vi "Senden-01-17.vi"(5 "error in":errorcluster, 6 "BefehlsCluster":T1, 7 "AbfragenCluster":cluster{string[], string[], string[]}, 8 "Abfragenr.Cluster":cluster{i32, i32, i32}, 9 "Senden?":bool[](array[boolean]), 10 "FPGA VI Reference In":refnum<k20>) -> (0 "BefehlsCluster":T1, 2 "error out":errorcluster, 3 "Senden?":bool[](array[boolean]), 4 "Abfragenr.Cluster":cluster{i32, i32, i32})   [LabVIEW 2010]
uses:
  <vilib>/rvi/interface/nirviMethod/nirviMethod.xnode
  C:/Users/HAGAR-IV/Desktop/Zeugs/markus/version feb 2012/FPGA Bitfiles/pertrasgcfpga2_FPGATarget_FPGA-Programm-01_A75D3647.lvbitx
  C:/Users/HAGAR-IV/Desktop/Zeugs/Johnny/pertrasgc fpga/FPGA-Programm-01-17.vi
  <vilib>/rvi/interface/common/niFpgaNodeNameForErrorReporting.ctl
  <vilib>/rvi/errors/niLvFpgaWhatHappensToTopLevelVI.ctl
  <vilib>/Utility/error.llb/Error Cluster From Error Code.vi
  <vilib>/rvi/errors/niLvFpgaAdjustHostInterfaceError.vi
  NiFpgaLv.dll
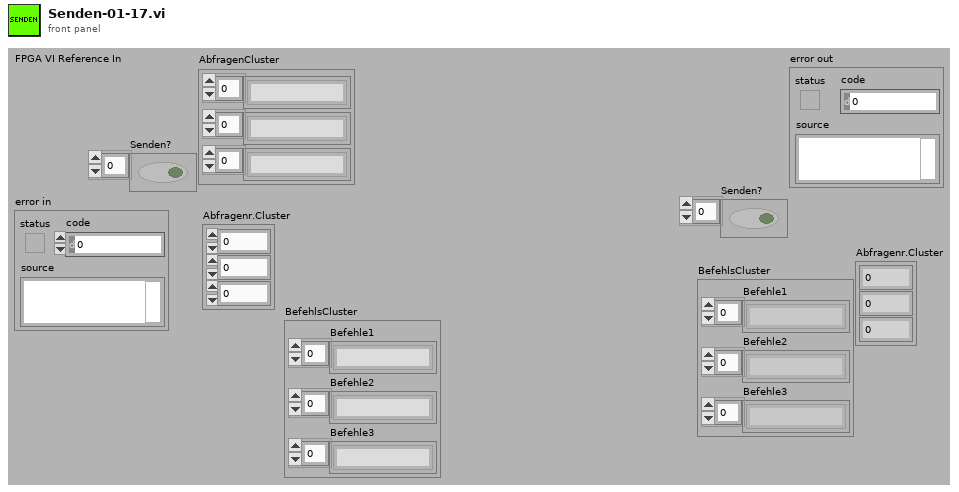
[diagram p1: front panel]
types:
  T1 = cluster{"Befehle1":string[], "Befehle2":string[], "Befehle3":string[]}
  T2 = typedef "niFpgaNodeNameForErrorReporting.ctl" = enum16{"Open FPGA VI Reference", "Read/Write Control", "Invoke Method: Abort", "Invoke Method: Acknowledge IRQ", "Invoke Method: Download", "Invoke Method: FIFO.Configure", "Invoke Method: FIFO.Read", "Invoke Method: FIFO.Start", "Invoke Method: FIFO.Stop", "Invoke Method: FIFO.Write", "Invoke Method: Reset", "Invoke Method: Run", "Invoke Method: Wait on IRQ", "Close FPGA VI Reference"}
  T3 = typedef "niLvFpgaWhatHappensToTopLevelVI.ctl" = enum16{"top level VI scripted behind XNode", "top level VI inlined behind XNode"}
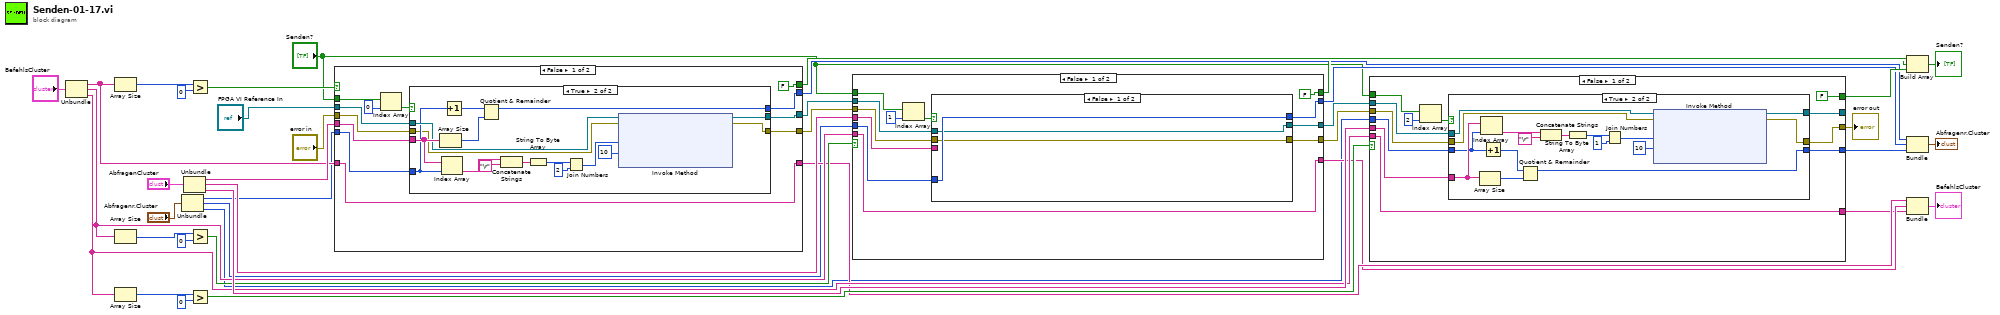
[diagram p0: block diagram]
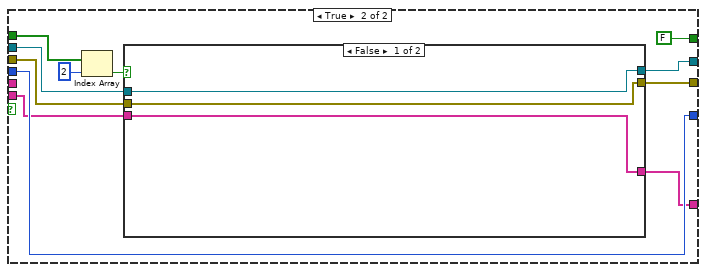
[diagram p3: hidden frame]
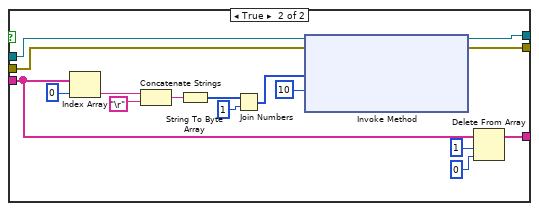
[diagram p4: hidden frame]
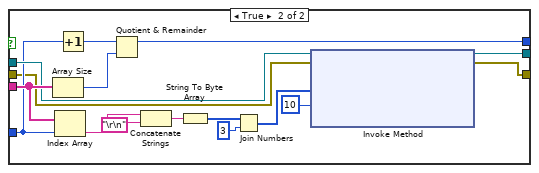
[diagram p5: hidden frame]
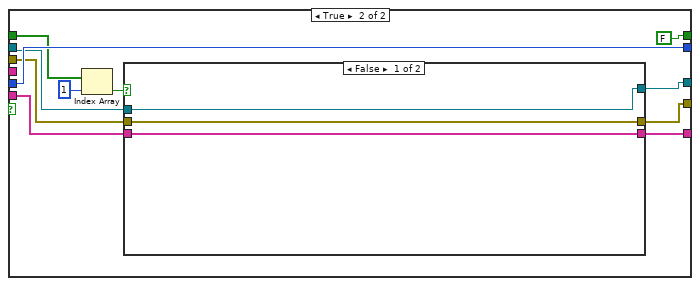
[diagram p6: hidden frame]
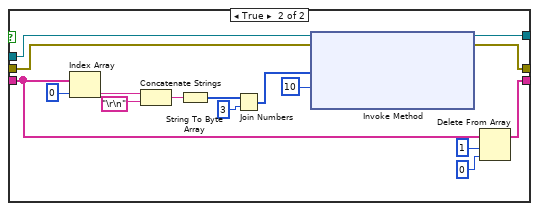
[diagram p7: hidden frame]
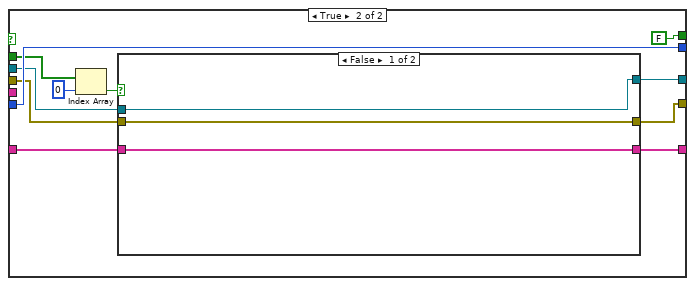
[diagram p9: hidden frame]
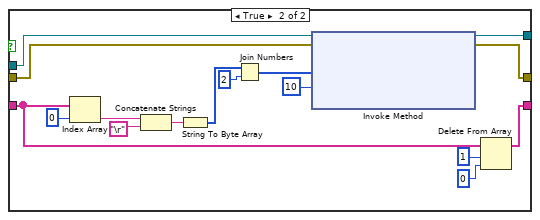
[diagram p10: hidden frame]
diagram:
  n1 = Unbundle("BefehlsCluster") -> ("Befehle1"=w26:string[], "Befehle2"=w25:string[], "Befehle3"=w24:string[])
  n2 = Array Size(array=w26) -> (size(s)=w41:i32)
  n3 = Array Size(array=w25) -> (size(s)=w35:i32)
  n4 = Array Size(array=w24) -> (size(s)=w32:i32)
  n5 = Unbundle("Abfragenr.Cluster") -> (w14:i32, w13:i32, w12:i32)
  n6 = Unbundle("AbfragenCluster") -> (w38:string[], w37:string[], w36:string[])
  n7 = Greater?(x=w41, y=0) -> (0:w39:bool)
  n8 = Greater?(x=w35, y=0) -> (0:w33:bool)
  n9 = Greater?(x=w32, y=0) -> (0:w30:bool)
  n10 = case shown="False" w39 {
    tunnel: w26 -> [w53 w146]
    tunnel: [w53 w145] -> w23
    tunnel: "Senden?" -> [w47 w143]
    tunnel: [FALSE FALSE] -> w19
    tunnel: w14 -> [w50 w149]
    tunnel: "FPGA VI Reference In" -> [w49 w144]
    tunnel: [w48 w149] -> w11
    tunnel: w38 -> [w46 _]
    tunnel: [w45 w142] -> w29
    tunnel: "error in" -> [w43 w140]
    tunnel: [w42 w139] -> w4
    frame False {
      n11 = Index Array(array=w47, index=0 ("Index")) -> (element=w51:bool)
      n12 = case shown="True" w51 {
        tunnel: w46 -> [_ w70]
        tunnel: w50 -> [w56 w64]
        tunnel: w49 -> [w55 w67]
        tunnel: [w56 w63] -> w48
        tunnel: [w55 w62] -> w45
        tunnel: w43 -> [w54 w58]
        tunnel: [w54 w57] -> w42
        frame False {
        }
        frame True {
          n13 = Array Size(array=w70) -> (size(s)=w71:i32)
          n14 = Index Array(array=w70, index=w64) -> (element=w60:string)
          n15 = Increment(x=w64) -> (x+1=w72:i32)
          n16 = Quotient & Remainder(x=w72, y=w71) -> (x-y*floor(x/y)=w63:i32)  [unwired: 1 out]
          n17 = Concatenate Strings(w60, "\r") -> (w61:string)
          n18 = String To Byte Array(string=w61) -> (unsigned byte array=w69:u8[])
          n19 = Join Numbers(hi=w69, lo=u8 2) -> ((hi.lo)=w66:u16[])
          n20 = xnode "Invoke Method"("FPGA VI Reference In"=w67, "error in"=w58, "Data"=w66, "Timeout (ms)"=10) -> ("FPGA VI Reference Out"=w62:refnum<k20>, "error out"=w57:errorcluster)  [unwired: 1 out]
        }
      }
    }
    frame True {
      n21 = Index Array(array=w143, index=0 ("Index")) -> (element=w147:bool)
      n22 = case shown="False" w147 {
        tunnel: w146 -> [w152 w164]
        tunnel: [w152 w166] -> w145
        tunnel: w144 -> [w151 w165]
        tunnel: [w151 w158] -> w142
        tunnel: w140 -> [w150 w154]
        tunnel: [w150 w153] -> w139
        frame False {
        }
        frame True {
          n23 = Index Array(array=w164, index=0 ("Index")) -> (element=w156:string)
          n24 = Concatenate Strings(w156, "\r") -> (w155:string)
          n25 = String To Byte Array(string=w155) -> (unsigned byte array=w162:u8[])
          n26 = Join Numbers(hi=w162, lo=u8 2) -> ((hi.lo)=w160:u16[])
          n27 = xnode "Invoke Method"("FPGA VI Reference In"=w165, "error in"=w154, "Data"=w160, "Timeout (ms)"=10) -> ("FPGA VI Reference Out"=w158:refnum<k20>, "error out"=w153:errorcluster)  [unwired: 1 out]
          n28 = Delete From Array(array=w164, length=1 ("Länge"), index=0 ("Index")) -> (array with subset deleted=w166:string[])  [unwired: 1 out]
        }
      }
    }
  }
  n29 = case shown="False" w33 {
    tunnel: w25 -> [w246 w339]
    tunnel: [w246 w338] -> w22
    tunnel: "Senden?" -> [w240 w336]
    tunnel: w13 -> [w243 w342]
    tunnel: w29 -> [w242 w337]
    tunnel: [w241 w342] -> w10
    tunnel: w37 -> [w239 _]
    tunnel: [w238 w335] -> w28
    tunnel: [FALSE FALSE] -> w17
    tunnel: w4 -> [w236 w333]
    tunnel: [w235 w332] -> w3
    frame False {
      n30 = Index Array(array=w240, index=1 ("Index")) -> (element=w244:bool)
      n31 = case shown="False" w244 {
        tunnel: w239 -> [_ w263]
        tunnel: w243 -> [w249 w257]
        tunnel: w242 -> [w248 w260]
        tunnel: [w249 w256] -> w241
        tunnel: [w248 w255] -> w238
        tunnel: w236 -> [w247 w251]
        tunnel: [w247 w250] -> w235
        frame False {
        }
        frame True {
          n32 = Array Size(array=w263) -> (size(s)=w264:i32)
          n33 = Index Array(array=w263, index=w257) -> (element=w253:string)
          n34 = Increment(x=w257) -> (x+1=w265:i32)
          n35 = Quotient & Remainder(x=w265, y=w264) -> (x-y*floor(x/y)=w256:i32)  [unwired: 1 out]
          n36 = Concatenate Strings(w253, "\r\n") -> (w252:string)
          n37 = String To Byte Array(string=w252) -> (unsigned byte array=w262:u8[])
          n38 = Join Numbers(hi=w262, lo=u8 3) -> ((hi.lo)=w259:u16[])
          n39 = xnode "Invoke Method"("FPGA VI Reference In"=w260, "error in"=w251, "Data"=w259, "Timeout (ms)"=10) -> ("FPGA VI Reference Out"=w255:refnum<k20>, "error out"=w250:errorcluster)  [unwired: 1 out]
        }
      }
    }
    frame True {
      n40 = Index Array(array=w336, index=1 ("Index")) -> (element=w340:bool)
      n41 = case shown="False" w340 {
        tunnel: w339 -> [w345 w357]
        tunnel: [w345 w359] -> w338
        tunnel: w337 -> [w344 w358]
        tunnel: [w344 w351] -> w335
        tunnel: w333 -> [w343 w347]
        tunnel: [w343 w346] -> w332
        frame False {
        }
        frame True {
          n42 = Index Array(array=w357, index=0 ("Index")) -> (element=w349:string)
          n43 = Concatenate Strings(w349, "\r\n") -> (w348:string)
          n44 = String To Byte Array(string=w348) -> (unsigned byte array=w355:u8[])
          n45 = Join Numbers(hi=w355, lo=u8 3) -> ((hi.lo)=w353:u16[])
          n46 = xnode "Invoke Method"("FPGA VI Reference In"=w358, "error in"=w347, "Data"=w353, "Timeout (ms)"=10) -> ("FPGA VI Reference Out"=w351:refnum<k20>, "error out"=w346:errorcluster)  [unwired: 1 out]
          n47 = Delete From Array(array=w357, length=1 ("Länge"), index=0 ("Index")) -> (array with subset deleted=w359:string[])  [unwired: 1 out]
        }
      }
    }
  }
  n48 = case shown="False" w30 {
    tunnel: w24 -> [w439 w532]
    tunnel: [w439 w531] -> w21
    tunnel: "Senden?" -> [w433 w529]
    tunnel: w12 -> [w436 w535]
    tunnel: w28 -> [w435 w530]
    tunnel: [w434 w535] -> w9
    tunnel: w36 -> [w432 _]
    tunnel: [FALSE FALSE] -> w16
    tunnel: [w430 w527] -> _
    tunnel: w3 -> [w429 w526]
    tunnel: [w428 w525] -> w2
    frame False {
      n49 = Index Array(array=w433, index=2 ("Index")) -> (element=w437:bool)
      n50 = case shown="True" w437 {
        tunnel: w432 -> [_ w456]
        tunnel: w436 -> [w442 w450]
        tunnel: w435 -> [w441 w453]
        tunnel: [w442 w449] -> w434
        tunnel: [w441 w448] -> w430
        tunnel: w429 -> [w440 w444]
        tunnel: [w440 w443] -> w428
        frame False {
        }
        frame True {
          n51 = Array Size(array=w456) -> (size(s)=w457:i32)
          n52 = Index Array(array=w456, index=w450) -> (element=w446:string)
          n53 = Increment(x=w450) -> (x+1=w458:i32)
          n54 = Quotient & Remainder(x=w458, y=w457) -> (x-y*floor(x/y)=w449:i32)  [unwired: 1 out]
          n55 = Concatenate Strings(w446, "\r") -> (w445:string)
          n56 = String To Byte Array(string=w445) -> (unsigned byte array=w455:u8[])
          n57 = Join Numbers(hi=w455, lo=u8 1) -> ((hi.lo)=w452:u16[])
          n58 = xnode "Invoke Method"("FPGA VI Reference In"=w453, "error in"=w444, "Data"=w452, "Timeout (ms)"=10) -> ("FPGA VI Reference Out"=w448:refnum<k20>, "error out"=w443:errorcluster)  [unwired: 1 out]
        }
      }
    }
    frame True {
      n59 = Index Array(array=w529, index=2 ("Index")) -> (element=w533:bool)
      n60 = case shown="False" w533 {
        tunnel: w532 -> [w538 w550]
        tunnel: [w538 w552] -> w531
        tunnel: w530 -> [w537 w551]
        tunnel: [w537 w544] -> w527
        tunnel: w526 -> [w536 w540]
        tunnel: [w536 w539] -> w525
        frame False {
        }
        frame True {
          n61 = Index Array(array=w550, index=0 ("Index")) -> (element=w542:string)
          n62 = Concatenate Strings(w542, "\r") -> (w541:string)
          n63 = String To Byte Array(string=w541) -> (unsigned byte array=w548:u8[])
          n64 = Join Numbers(hi=w548, lo=u8 1) -> ((hi.lo)=w546:u16[])
          n65 = xnode "Invoke Method"("FPGA VI Reference In"=w551, "error in"=w540, "Data"=w546, "Timeout (ms)"=10) -> ("FPGA VI Reference Out"=w544:refnum<k20>, "error out"=w539:errorcluster)  [unwired: 1 out]
          n66 = Delete From Array(array=w550, length=1 ("Länge"), index=0 ("Index")) -> (array with subset deleted=w552:string[])  [unwired: 1 out]
        }
      }
    }
  }
  "error out" <- w2
  n67 = Build Array(w19, w17, w16) -> (→"Senden?":bool[])
  n68 = Bundle(w11, w10, w9) -> (→"Abfragenr.Cluster":cluster{i32, i32, i32})  [unwired: 1 in]
  n69 = Bundle("Befehle1"=w23, "Befehle2"=w22, "Befehle3"=w21) -> (→"BefehlsCluster":T1)  [unwired: 1 in]
